vi "Calc Mean.vi"(11 "JSON Object In":refnum<class "JSON Object.lvclass">) -> (3 "JSON Value":refnum<class "JSON Value.lvclass">)   [LabVIEW 2020, in "Library Commun.lvlib" / "JSON Object.lvclass"]
uses:
  JSON Object.lvclass
  C:/Users/ngarcin/OneDrive - Altyor/Standard TB/Class/JSON API/JSON Value/JSON Value.lvclass
  JSON Value/JSON Value.lvclass
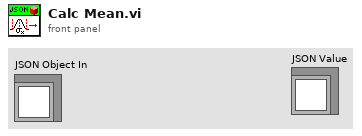
[diagram p1: front panel]
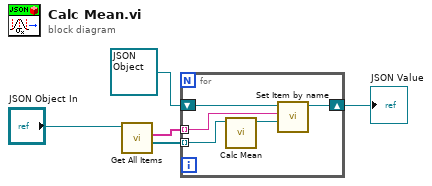
[diagram p0: block diagram]
diagram:
  n1 = call-dynamic "Get All Items.vi"("JSON Object in"="JSON Object In") -> ("Values"=w4:refnum<class "JSON Value.lvclass">[], "Item Names"=w3:string[])  [unwired: 7 in, 2 out]
  n2 = for {
    tunnel: w4 -> [w10] mode=indexing
    tunnel: w3 -> [w8] mode=indexing
    shift-right: [w6] -> w1
    shift-left: refnum<class "JSON Object.lvclass"> refnum ("JSON Object In") -> [w9]
    n3 = call-dynamic "Calc Mean.vi"("JSON Value In"=w10) -> ("JSON Value"=w7:refnum<class "JSON Value.lvclass">)  [unwired: 10 in]
    n4 = call-dynamic "Set Item by name.vi"("Value"=w7, "name"=w8, "JSON Object in"=w9) -> ("JSON Object out"=w6:refnum<class "JSON Object.lvclass">)  [unwired: 6 in, 2 out]
  }
  "JSON Value" <- w1
